vi "DataManagementGetDataSetsRequest_Parse.vi"(8 "error in (no error)":errorcluster, 11 "Message":T8) -> (0 "error out":errorcluster, 1 "Body":T1, 2 "Header":T7, 3 "DataManagementGetDataSetsRequest":T6)   [LabVIEW 2017]
uses:
  <vilib>/addons/InsightCM/MessageBus/Base/controls/Message.ctl
  <vilib>/addons/InsightCM/MessageBus/Base/controls/MessageHeader.ctl
  <vilib>/addons/InsightCM/MessageBus/Base/controls/KeyValuePair.ctl
  <vilib>/addons/InsightCM/MessageBus/MessageLibrary/DataManagement/controls/DataManagementGetDataSetsRequest.ctl
  <vilib>/addons/InsightCM/MessageBus/MessageLibrary/DataManagement/controls/DataManagementGetDataSetsRequestBody.ctl
  <vilib>/addons/InsightCM/MessageBus/Base/controls/DataSetQueryParams.ctl
  <vilib>/addons/InsightCM/MessageBus/Base/controls/TrendPoint.ctl
  <vilib>/addons/InsightCM/MessageBus/Base/controls/DataSetProcessing.ctl
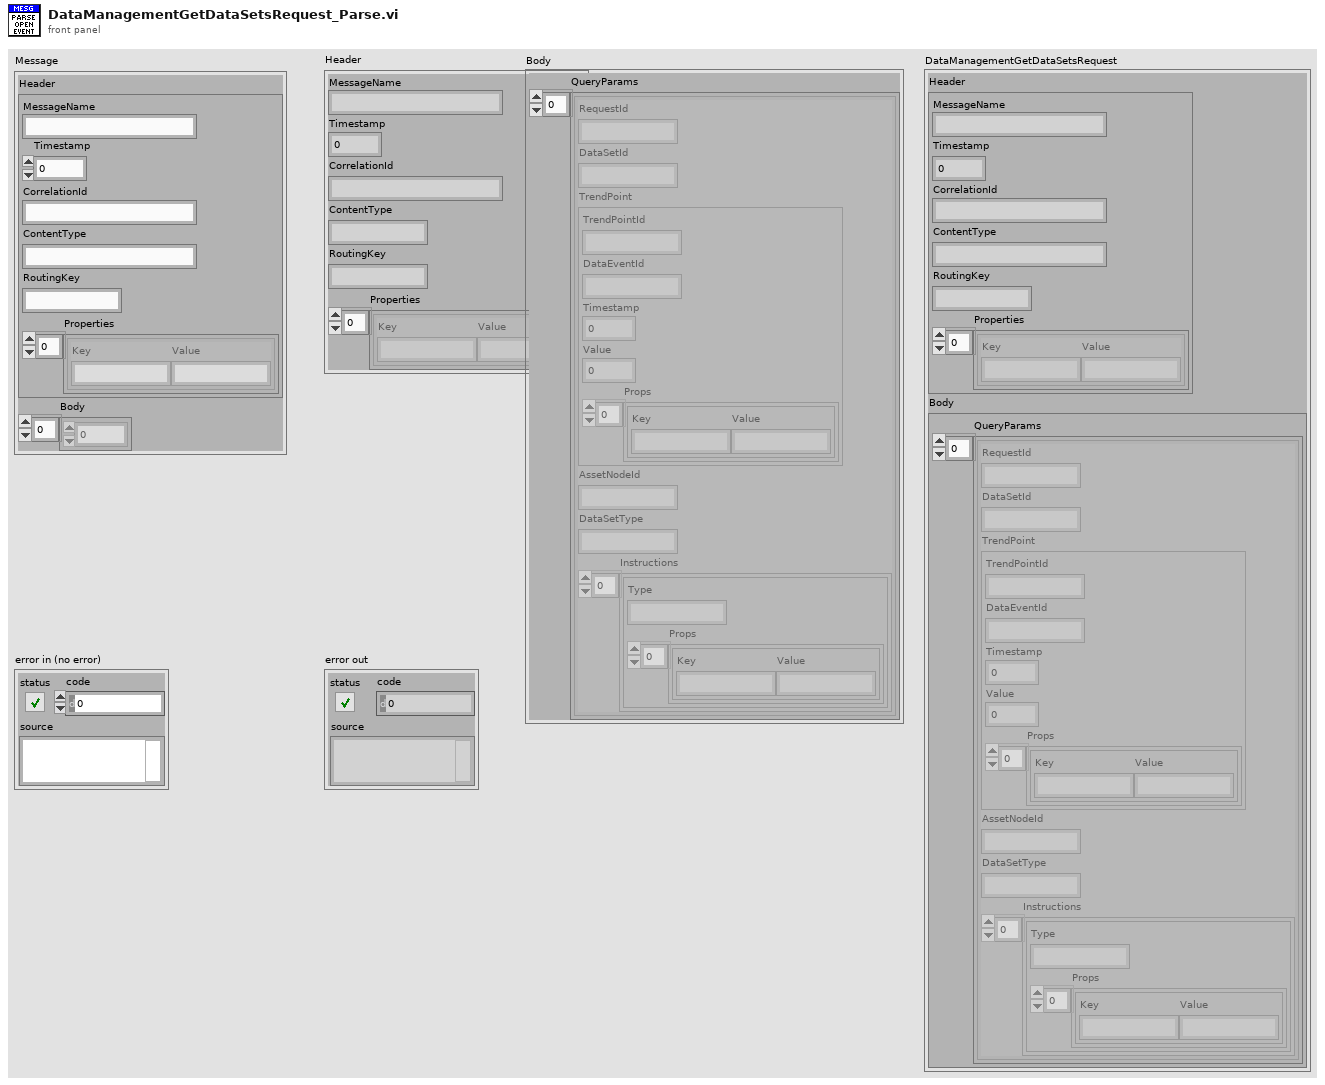
[diagram p1: front panel]
types:
  T1 = typedef "DataManagementGetDataSetsRequestBody.ctl" = cluster{"QueryParams":T2[]}
  T2 = typedef "DataSetQueryParams.ctl" = cluster{"RequestId":string, "DataSetId":string, "TrendPoint":T3, "AssetNodeId":string, "DataSetType":string, "Instructions":T5[]}
  T3 = typedef "TrendPoint.ctl" = cluster{"TrendPointId":string, "DataEventId":string, "Timestamp":i64, "Value":dbl, "Props":T4[]}
  T4 = typedef "KeyValuePair.ctl" = cluster{"Key":string, "Value":string}
  T5 = typedef "DataSetProcessing.ctl" = cluster{"Type":string, "Props":T4[]}
  T6 = typedef "DataManagementGetDataSetsRequest.ctl" = cluster{"Header":T7, "Body":T1}
  T7 = typedef "MessageHeader.ctl" = cluster{"MessageName":string, "Timestamp":i64, "CorrelationId":string, "ContentType":string, "RoutingKey":string, "Properties":T4[]}
  T8 = typedef "Message.ctl" = cluster{"Header":T7, "Body":u8[]}
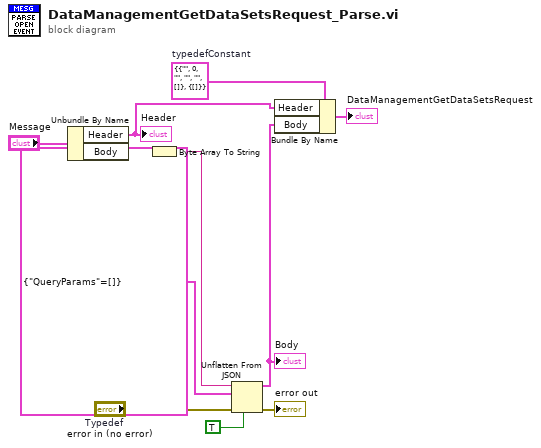
[diagram p0: block diagram]
diagram:
  w3 = T6 {"Header"={"MessageName"="", "Timestamp"=0, "CorrelationId"="", "ContentType"="", "RoutingKey"="", "Properties"=[]}, "Body"={"QueryParams"=[]}}  # typedefConstant
  w7 = T1 {"QueryParams"=[]}  # Typedef
  n1 = Unbundle By Name("Message") -> ("Header"=w9:T7, "Body"=w1:u8[])
  "Header" <- w9
  n2 = Byte Array To String(unsigned byte array=w1) -> (string=w6:string)
  n3 = Unflatten From JSON(JSON string=w6, type and defaults=w7, default null elements? (F)=TRUE, error in (no error)="error in (no error)") -> (value=w5:T1, error out=→"error out":errorcluster)  [unwired: 3 in]
  "Body" <- w5
  n4 = Bundle By Name(cluster=w3, "Header"=w9, "Body"=w5) -> (→"DataManagementGetDataSetsRequest":T6)
